vi "stop.vi"(8 "error in (no error)":errorcluster, 10 "stop?":bool, 11 "DDSOutput in":refnum<class "DDSOutput.lvclass">) -> (0 "error out":errorcluster, 2 "hasStopped":bool, 3 "DDSOutput out":refnum<class "DDSOutput.lvclass">)   [LabVIEW 2011, in "Hardware.lvlib" / "Channels.lvlib" / "DDSOutput.lvclass"]
uses:
  DDSOutput.lvclass
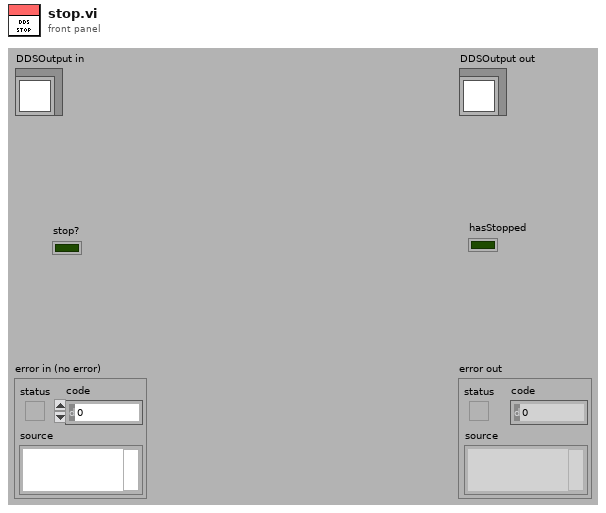
[diagram p1: front panel]
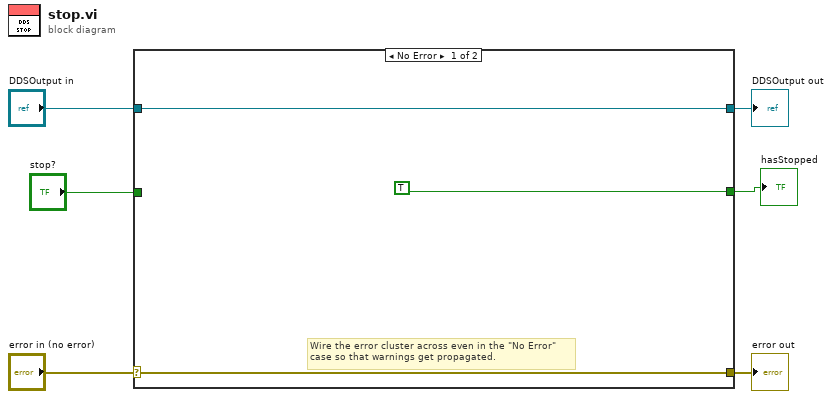
[diagram p0: block diagram]
diagram:
  n1 = case shown="No Error" "error in (no error)" {
    selector: "error in (no error)" -> [w8 w11]
    tunnel: [w8 w11] -> w5
    tunnel: [w9 w10] -> w3
    tunnel: "DDSOutput in" -> [w9 w10]
    tunnel: "stop?" -> [_ _]
    tunnel: [TRUE _] -> w1
    frame No Error {
      # "Wire the error cluster across even in the \"No Error\"\ncase so that warnings get propagated."
    }
    frame Error {
    }
  }
  "error out" <- w5
  "DDSOutput out" <- w3
  "hasStopped" <- w1
